vi "Average RF Traces.vi"(8 "error in (no error)":errorcluster, 9 "RF Traces In":waveform(dbl)[][](array[waveform]), 10 "Filter":T1={"Upper Cutoff [Hz]"=10000000.0, "Lower Cutoff [Hz]"=1000000.0, "Order"=2, "Type"=enum."No Filter"} {"Upper Cutoff [Hz]" min=100000.0 max=100000000.0 step=100000.0 format="%#_6p"; "Lower Cutoff [Hz]" min=100000.0 max=100000000.0 step=100000.0 format="%#_6p"}) -> (0 "error out":errorcluster, 1 "Averaged Traces Out":waveform(dbl)[](array[waveform]))   [LabVIEW 2019]
uses:
  RF Filter Control.ctl
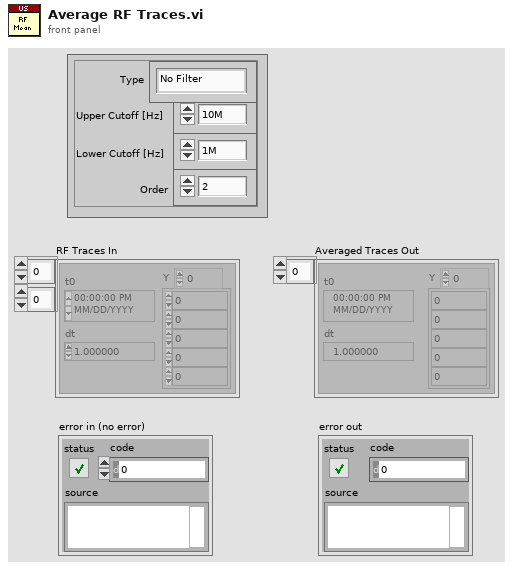
[diagram p1: front panel]
types:
  T1 = typedef "RF Filter Control.ctl" = cluster{"Upper Cutoff [Hz]":dbl, "Lower Cutoff [Hz]":dbl, "Order":i32, "Type":enum16{"Bandpass", "AC", "No Filter"}}
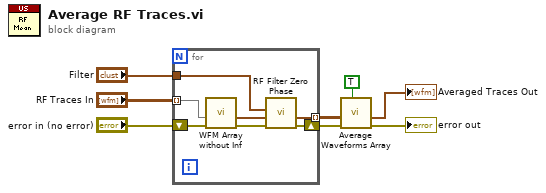
[diagram p0: block diagram]
diagram:
  n1 = for {
    tunnel: [w15] -> w4 mode=indexing
    tunnel: "Filter" -> [w13]
    shift-right: [w10] -> w3
    shift-left: "error in (no error)" -> [w11]
    tunnel: "RF Traces In" -> [w9] mode=indexing
    n2 = call "WFM Array without Inf.vi"("Error In"=w11, "Waveforms in"=w9) -> ("Error Out"=w12:errorcluster, "Waveforms Out"=w14:waveform(dbl)[])  [unwired: 8 in]
    n3 = call "RF Filter Zero Phase.vi"("Error In"=w12, "RF Signals In"=w14, "Filter Definition"=w13) -> ("Error Out"=w10:errorcluster, "Filtered RF Signals"=w15:waveform(dbl)[])  [unwired: 7 in]
  }
  n4 = call "Average Waveforms Array.vi"("Transpose?"=TRUE, "Error In"=w3, "Waveforms In"=w4) -> ("Error Out"=→"error out":errorcluster, "Averaged Waveforms"=→"Averaged Traces Out":waveform(dbl)[])  [unwired: 7 in]
